vi "set Packet Timeout M Sec.vi"(8 "error in (no error)":errorcluster, 10 "msec":dbl, 11 "port_num":i32) -> (0 "error out":errorcluster)   [LabVIEW 2022 SP3, in "dxl.lvlib"]
doc: "WINDECLSPEC void setPacketTimeoutMSec (int port_num, double msec);"
uses:
  dxl.lvlib
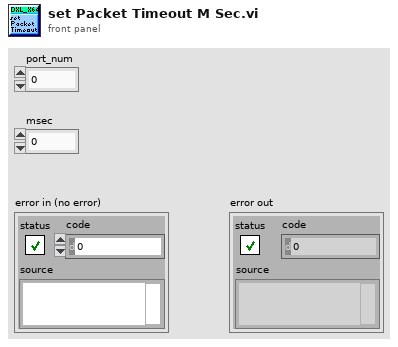
[diagram p1: front panel]
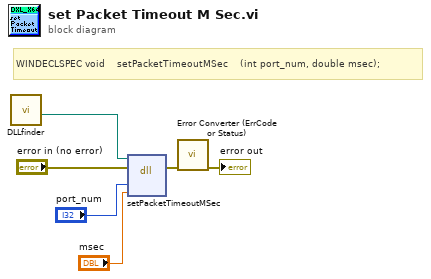
[diagram p0: block diagram]
diagram:
  # "WINDECLSPEC void    setPacketTimeoutMSec    (int port_num, double msec);"
  n1 = call "DLLfinder.vi"() -> ("File Path"=w1:path)  [unwired: 11 in]
  n2 = dll-call lib="C:/EnFlo_Software/ADAM Serial/Instrument drivers/Dynamixel/2nd attempt/Library/dxl_x64_c.*" fn="setPacketTimeoutMSec"(path in=w1, error in="error in (no error)", "port_num"="port_num", "msec"="msec") -> (error out=w3:errorcluster)  [unwired: 4 in, 1 out]
  n3 = call "Error Converter (ErrCode or Status).vi"("error in (no error)"=w3) -> ("error out"=→"error out":errorcluster)  [unwired: 10 in]
